vi "Write Data to TDMS File.vi"(8 "error in (no error)":errorcluster, 10 "TDMS-Container":refnum<class "TDMS-Container.lvclass">, 11 "TDMS-Actor in":refnum<class "TDMS-Actor.lvclass">) -> (0 "error out":errorcluster, 3 "TDMS-Actor out":refnum<class "TDMS-Actor.lvclass">)   [LabVIEW 2017, in "BNT_TDMS.lvlib" / "TDMS-Actor.lvclass"]
doc: "Write TDMS-Container to file and optionally change file."
uses:
  TDMS-Actor.lvclass
  TDMSContainer/TDMS-Container.lvclass
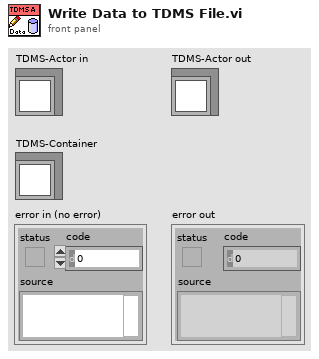
[diagram p1: front panel]
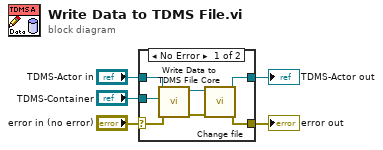
[diagram p0: block diagram]
diagram:
  n1 = case shown="No Error" "error in (no error)" {
    selector: "error in (no error)" -> [w11 w14]
    tunnel: [w6 w14] -> w4
    tunnel: [w8 w13] -> w2
    tunnel: "TDMS-Actor in" -> [w12 w13]
    tunnel: "TDMS-Container" -> [w10 _]
    frame No Error {
      n2 = call-dynamic "Write Data to TDMS File Core.vi"("error in (no error)"=w11, "TDMS-Container"=w10, "TDMS-Actor in"=w12) -> ("error out"=w7:errorcluster, "TDMS-Actor out"=w9:refnum<class "TDMS-Actor.lvclass">)  [unwired: 7 in]
      n3 = call "Change file.vi"("Error In"=w7, "TDMS-Actor in"=w9) -> ("Error Out"=w6:errorcluster, "TDMS-Actor out"=w8:refnum<class "TDMS-Actor.lvclass">)  [unwired: 8 in]
    }
    frame Error {
    }
  }
  "error out" <- w4
  "TDMS-Actor out" <- w2
